vi "WebView2 Viewer.vi"(2 "ProjectRef":refnum<vi>, 4 "Extra Scripts":string, 5 "FileDependency In":map{path, T1}(c390), 6 "Options":string, 7 "OpenWebBrowser(False)":bool, 8 "error in":errorcluster, 9 "Embedd VISJS Librarya in HTMl File(False)":bool, 10 "HTMLFilePath":path, 11 "LibraryDependency":map{path, T3}(c390)) -> (0 "error out":errorcluster, 3 "HTMLFileContent":string)   [LabVIEW 2020, in "WebView2-Viewer.lvlib"] (continued)
break}for(C||(C={id:t.id},g.node&&(C.attr=Yv(C.attr,g.node))),A=I.length-1;A>=0;A--){var o,n=I[A];n.nodes||(n.nodes=[]),-1===Xc(o=n.nodes).call(o,C)&&n.nodes.push(C)}t.attr&&(C.attr=Yv(C.attr,t.attr))}function Uv(g,t){if(g.edges||(g.edges=[]),g.edges.push(t),g.edge){var A=Yv({},g.edge);t.attr=Yv(A,t.attr)}}function _v(g,t,A,e,C){var I={from:t,to:A,type:e};return g.edge&&(I.attr=Yv({},g.edge)),I.attr=Yv(I.attr||{},C),null!=C&&C.hasOwnProperty(\"arrows\")&&null!=C.arrows&&(I.arrows={to:{enabled:!0,type:C.arrows.type}},C.arrows=null),I}function Kv(){for(Gv=Mv.NULL,Fv=\"\";\" \"===Zv||\"\\t\"===Zv||\"\\n\"===Zv||\"\\r\"===Zv;)jv();do{var g=!1;if(\"#\"===Zv){for(var t=Sv-1;\" \"===zv.charAt(t)||\"\\t\"===zv.charAt(t);)t--;if(\"\\n\"===zv.charAt(t)||\"\"===zv.charAt(t)){for(;\"\"!=Zv&&\"\\n\"!=Zv;)jv();g=!0}}if(\"/\"===Zv&&\"/\"===Lv()){for(;\"\"!=Zv&&\"\\n\"!=Zv;)jv();g=!0}if(\"/\"===Zv&&\"*\"===Lv()){for(;\"\"!=Zv;){if(\"*\"===Zv&&\"/\"===Lv()){jv(),jv();break}jv()}g=!0}for(;\" \"===Zv||\"\\t\"===Zv||\"\\n\"===Zv||\"\\r\"===Zv;)jv()}while(g);if(\"\"!==Zv){var A=Zv+Lv();if(Bv[A])return Gv=Mv.DELIMITER,Fv=A,jv(),void jv();if(Bv[Zv])return Gv=Mv.DELIMITER,Fv=Zv,void jv();if(Vv(Zv)||\"-\"===Zv){for(Fv+=Zv,jv();Vv(Zv);)Fv+=Zv,jv();return\"false\"===Fv?Fv=!1:\"true\"===Fv?Fv=!0:isNaN(Number(Fv))||(Fv=Number(Fv)),void(Gv=Mv.IDENTIFIER)}if('\"'===Zv){for(jv();\"\"!=Zv&&('\"'!=Zv||'\"'===Zv&&'\"'===Lv());)'\"'===Zv?(Fv+=Zv,jv()):\"\\\\\"===Zv&&\"n\"===Lv()?(Fv+=\"\\n\",jv()):Fv+=Zv,jv();if('\"'!=Zv)throw gy('End of string \" expected');return jv(),void(Gv=Mv.IDENTIFIER)}for(Gv=Mv.UNKNOWN;\"\"!=Zv;)Fv+=Zv,jv();throw new SyntaxError('Syntax error in part \"'+ty(Fv,30)+'\"')}Gv=Mv.DELIMITER}function Hv(g){for(;\"\"!==Fv&&\"}\"!=Fv;)Xv(g),\";\"===Fv&&Kv()}function Xv(g){var t=Jv(g);if(t)qv(g,t);else{var A=function(g){if(\"node\"===Fv)return Kv(),g.node=$v(),\"node\";if(\"edge\"===Fv)return Kv(),g.edge=$v(),\"edge\";if(\"graph\"===Fv)return Kv(),g.graph=$v(),\"graph\";return null}(g);if(!A){if(Gv!=Mv.IDENTIFIER)throw gy(\"Identifier expected\");var e=Fv;if(Kv(),\"=\"===Fv){if(Kv(),Gv!=Mv.IDENTIFIER)throw gy(\"Identifier expected\");g[e]=Fv,Kv()}else!function(g,t){var A={id:t},e=$v();e&&(A.attr=e);Qv(g,A),qv(g,t)}(g,e)}}}function Jv(g){var t=null;if(\"subgraph\"===Fv&&((t={}).type=\"subgraph\",Kv(),Gv===Mv.IDENTIFIER&&(t.id=Fv,Kv())),\"{\"===Fv){if(Kv(),t||(t={}),t.parent=g,t.node=g.node,t.edge=g.edge,t.graph=g.graph,Hv(t),\"}\"!=Fv)throw gy(\"Angle bracket } expected\");Kv(),delete t.node,delete t.edge,delete t.graph,delete t.parent,g.subgraphs||(g.subgraphs=[]),g.subgraphs.push(t)}return t}function qv(g,t){for(;\"->\"===Fv||\"--\"===Fv;){var A,e=Fv;Kv();var C=Jv(g);if(C)A=C;else{if(Gv!=Mv.IDENTIFIER)throw gy(\"Identifier or subgraph expected\");Qv(g,{id:A=Fv}),Kv()}Uv(g,_v(g,t,A,e,$v())),t=A}}function $v(){for(var g,t,A=null,e={dashed:!0,solid:!1,dotted:[1,5]},C={dot:\"circle\",box:\"box\",crow:\"crow\",curve:\"curve\",icurve:\"inv_curve\",normal:\"triangle\",inv:\"inv_triangle\",diamond:\"diamond\",tee:\"bar\",vee:\"vee\"},I=new Array,i=new Array;\"[\"===Fv;){for(Kv(),A={};\"\"!==Fv&&\"]\"!=Fv;){if(Gv!=Mv.IDENTIFIER)throw gy(\"Attribute name expected\");var o=Fv;if(Kv(),\"=\"!=Fv)throw gy(\"Equal sign = expected\");if(Kv(),Gv!=Mv.IDENTIFIER)throw gy(\"Attribute value expected\");var n=Fv;\"style\"===o&&(n=e[n]),\"arrowhead\"===o&&(o=\"arrows\",n={to:{enabled:!0,type:C[n]}}),\"arrowtail\"===o&&(o=\"arrows\",n={from:{enabled:!0,type:C[n]}}),I.push({attr:A,name:o,value:n}),i.push(o),Kv(),\",\"==Fv&&Kv()}if(\"]\"!=Fv)throw gy(\"Bracket ] expected\");Kv()}if(Ic(i).call(i,\"dir\")){var r={arrows:{}};for(g=0;g<I.length;g++)if(\"arrows\"===I[g].name)if(null!=I[g].value.to)r.arrows.to=g;else{if(null==I[g].value.from)throw gy(\"Invalid value of arrows\");r.arrows.from=g}else\"dir\"===I[g].name&&(r.dir=g);var s,a,d=I[r.dir].value;if(!Ic(i).call(i,\"arrows\"))if(\"both\"===d)I.push({attr:I[r.dir].attr,name:\"arrows\",value:{to:{enabled:!0}}}),r.arrows.to=I.length-1,I.push({attr:I[r.dir].attr,name:\"arrows\",value:{from:{enabled:!0}}}),r.arrows.from=I.length-1;else if(\"forward\"===d)I.push({attr:I[r.dir].attr,name:\"arrows\",value:{to:{enabled:!0}}}),r.arrows.to=I.length-1;else if(\"back\"===d)I.push({attr:I[r.dir].attr,name:\"arrows\",value:{from:{enabled:!0}}}),r.arrows.from=I.length-1;else{if(\"none\"!==d)throw gy('Invalid dir type \"'+d+'\"');I.push({attr:I[r.dir].attr,name:\"arrows\",value:\"\"}),r.arrows.to=I.length-1}if(\"both\"===d)r.arrows.to&&r.arrows.from?(a=I[r.arrows.to].value.to.type,s=I[r.arrows.from].value.from.type,I[r.arrows.to]={attr:I[r.arrows.to].attr,name:I[r.arrows.to].name,value:{to:{enabled:!0,type:a},from:{enabled:!0,type:s}}},Zl(I).call(I,r.arrows.from,1)):r.arrows.to?(a=I[r.arrows.to].value.to.type,s=\"arrow\",I[r.arrows.to]={attr:I[r.arrows.to].attr,name:I[r.arrows.to].name,value:{to:{enabled:!0,type:a},from:{enabled:!0,type:s}}}):r.arrows.from&&(a=\"arrow\",s=I[r.arrows.from].value.from.type,I[r.arrows.from]={attr:I[r.arrows.from].attr,name:I[r.arrows.from].name,value:{to:{enabled:!0,type:a},from:{enabled:!0,type:s}}});else if(\"back\"===d)r.arrows.to&&r.arrows.from?(a=\"\",s=I[r.arrows.from].value.from.type,I[r.arrows.from]={attr:I[r.arrows.from].attr,name:I[r.arrows.from].name,value:{to:{enabled:!0,type:a},from:{enabled:!0,type:s}}}):r.arrows.to?(a=\"\",s=\"arrow\",r.arrows.from=r.arrows.to,I[r.arrows.from]={attr:I[r.arrows.from].attr,name:I[r.arrows.from].name,value:{to:{enabled:!0,type:a},from:{enabled:!0,type:s}}}):r.arrows.from&&(a=\"\",s=I[r.arrows.from].value.from.type,I[r.arrows.to]={attr:I[r.arrows.from].attr,name:I[r.arrows.from].name,value:{to:{enabled:!0,type:a},from:{enabled:!0,type:s}}}),I[r.arrows.from]={attr:I[r.arrows.from].attr,name:I[r.arrows.from].name,value:{from:{enabled:!0,type:I[r.arrows.from].value.from.type}}};else if(\"none\"===d){var h;I[h=r.arrows.to?r.arrows.to:r.arrows.from]={attr:I[h].attr,name:I[h].name,value:\"\"}}else{if(\"forward\"!==d)throw gy('Invalid dir type \"'+d+'\"');r.arrows.to&&r.arrows.from||r.arrows.to?(a=I[r.arrows.to].value.to.type,s=\"\",I[r.arrows.to]={attr:I[r.arrows.to].attr,name:I[r.arrows.to].name,value:{to:{enabled:!0,type:a},from:{enabled:!0,type:s}}}):r.arrows.from&&(a=\"arrow\",s=\"\",r.arrows.to=r.arrows.from,I[r.arrows.to]={attr:I[r.arrows.to].attr,name:I[r.arrows.to].name,value:{to:{enabled:!0,type:a},from:{enabled:!0,type:s}}}),I[r.arrows.to]={attr:I[r.arrows.to].attr,name:I[r.arrows.to].name,value:{to:{enabled:!0,type:I[r.arrows.to].value.to.type}}}}Zl(I).call(I,r.dir,1)}if(Ic(i).call(i,\"penwidth\")){var l=[];for(t=I.length,g=0;g<t;g++)\"width\"!==I[g].name&&(\"penwidth\"===I[g].name&&(I[g].name=\"width\"),l.push(I[g]));I=l}for(t=I.length,g=0;g<t;g++)Wv(I[g].attr,I[g].name,I[g].value);return A}function gy(g){return new SyntaxError(g+', got \"'+ty(Fv,30)+'\" (char '+Sv+\")\")}function ty(g,t){return g.length<=t?g:g.substr(0,27)+\"...\"}function Ay(g,t,A){for(var e=t.split(\".\"),C=e.pop(),I=g,i=0;i<e.length;i++){var o=e[i];o in I||(I[o]={}),I=I[o]}return I[C]=A,g}function ey(g,t){var A={};for(var e in g)if(g.hasOwnProperty(e)){var C=t[e];Rh(C)?Cl(C).call(C,(function(t){Ay(A,t,g[e])})):Ay(A,\"string\"==typeof C?C:e,g[e])}return A}function Cy(g){var t,A=Nv(g),e={nodes:[],edges:[],options:{}};A.nodes&&Cl(t=A.nodes).call(t,(function(g){var t={id:g.id,label:String(g.label||g.id)};Yv(t,ey(g.attr,Rv)),t.image&&(t.shape=\"image\"),e.nodes.push(t)}));if(A.edges){var C,I=function(g){var t={from:g.from,to:g.to};return Yv(t,ey(g.attr,Pv)),null==t.arrows&&\"->\"===g.type&&(t.arrows=\"to\"),t};Cl(C=A.edges).call(C,(function(g){var t,A,C,i,o,n,r;(t=g.from instanceof Object?g.from.nodes:{id:g.from},A=g.to instanceof Object?g.to.nodes:{id:g.to},g.from instanceof Object&&g.from.edges)&&Cl(C=g.from.edges).call(C,(function(g){var t=I(g);e.edges.push(t)}));(o=A,n=function(t,A){var C=_v(e,t.id,A.id,g.type,g.attr),i=I(C);e.edges.push(i)},Rh(i=t)?Cl(i).call(i,(function(g){Rh(o)?Cl(o).call(o,(function(t){n(g,t)})):n(g,o)})):Rh(o)?Cl(o).call(o,(function(g){n(i,g)})):n(i,o),g.to instanceof Object&&g.to.edges)&&Cl(r=g.to.edges).call(r,(function(g){var t=I(g);e.edges.push(t)}))}))}return A.attr&&(e.options=A.attr),e}var Iy=Object.freeze({__proto__:null,DOTToGraph:Cy,parseDOT:Nv});function iy(g,t){var A,e={edges:{inheritColor:!1},nodes:{fixed:!1,parseColor:!1}};null!=t&&(null!=t.fixed&&(e.nodes.fixed=t.fixed),null!=t.parseColor&&(e.nodes.parseColor=t.parseColor),null!=t.inheritColor&&(e.edges.inheritColor=t.inheritColor));var C=g.edges,I=Fh(C).call(C,(function(g){var t={from:g.source,id:g.id,to:g.target};return null!=g.attributes&&(t.attributes=g.attributes),null!=g.label&&(t.label=g.label),null!=g.attributes&&null!=g.attributes.title&&(t.title=g.attributes.title),\"Directed\"===g.type&&(t.arrows=\"to\"),g.color&&!1===e.edges.inheritColor&&(t.color=g.color),t}));return{nodes:Fh(A=g.nodes).call(A,(function(g){var t={id:g.id,fixed:e.nodes.fixed&&null!=g.x&&null!=g.y};return null!=g.attributes&&(t.attributes=g.attributes),null!=g.label&&(t.label=g.label),null!=g.size&&(t.size=g.size),null!=g.attributes&&null!=g.attributes.title&&(t.title=g.attributes.title),null!=g.title&&(t.title=g.title),null!=g.x&&(t.x=g.x),null!=g.y&&(t.y=g.y),null!=g.color&&(!0===e.nodes.parseColor?t.color=g.color:t.color={background:g.color,border:g.color,highlight:{background:g.color,border:g.color},hover:{background:g.color,border:g.color}}),t})),edges:I}}var oy=Object.freeze({__proto__:null,parseGephi:iy}),ny=Object.freeze({__proto__:null,cn:{addDescription:\"???????????\",addEdge:\"?????\",addNode:\"????\",back:\"??\",close:\"??\",createEdgeError:\"????????????\",del:\"????\",deleteClusterError:\"???????\",edgeDescription:\"??????????????????????????\",edit:\"??\",editClusterError:\"???????\",editEdge:\"?????\",editEdgeDescription:\"??????????????????\",editNode:\"????\"},cs:{addDescription:\"Kluknutím do prázdného prostoru mužete pridat nový vrchol.\",addEdge:\"Pridat hranu\",addNode:\"Pridat vrchol\",back:\"Zpet\",close:\"Zavrít\",createEdgeError:\"Nelze pripojit hranu ke shluku.\",del:\"Smazat výber\",deleteClusterError:\"Nelze mazat shluky.\",edgeDescription:\"Pretažením z jednoho vrcholu do druhého mužete spojit tyto vrcholy novou hranou.\",edit:\"Upravit\",editClusterError:\"Nelze upravovat shluky.\",editEdge:\"Upravit hranu\",editEdgeDescription:\"Pretažením kontrolního vrcholu hrany ji mužete pripojit k jinému vrcholu.\",editNode:\"Upravit vrchol\"},de:{addDescription:\"Klicke auf eine freie Stelle, um einen neuen Knoten zu plazieren.\",addEdge:\"Kante hinzufügen\",addNode:\"Knoten hinzufügen\",back:\"Zurück\",close:\"Schließen\",createEdgeError:\"Es ist nicht möglich, Kanten mit Clustern zu verbinden.\",del:\"Lösche Auswahl\",deleteClusterError:\"Cluster können nicht gelöscht werden.\",edgeDescription:\"Klicke auf einen Knoten und ziehe die Kante zu einem anderen Knoten, um diese zu verbinden.\",edit:\"Editieren\",editClusterError:\"Cluster können nicht editiert werden.\",editEdge:\"Kante editieren\",editEdgeDescription:\"Klicke auf die Verbindungspunkte und ziehe diese auf einen Knoten, um sie zu verbinden.\",editNode:\"Knoten editieren\"},en:{addDescription:\"Click in an empty space to place a new node.\",addEdge:\"Add Edge\",addNode:\"Add Node\",back:\"Back\",close:\"Close\",createEdgeError:\"Cannot link edges to a cluster.\",del:\"Delete selected\",deleteClusterError:\"Clusters cannot be deleted.\",edgeDescription:\"Click on a node and drag the edge to another node to connect them.\",edit:\"Edit\",editClusterError:\"Clusters cannot be edited.\",editEdge:\"Edit Edge\",editEdgeDescription:\"Click on the control points and drag them to a node to connect to it.\",editNode:\"Edit Node\"},es:{addDescription:\"Haga clic en un lugar vacío para colocar un nuevo nodo.\",addEdge:\"Añadir arista\",addNode:\"Añadir nodo\",back:\"Atrás\",close:\"Cerrar\",createEdgeError:\"No se puede conectar una arista a un grupo.\",del:\"Eliminar selección\",deleteClusterError:\"No es posible eliminar grupos.\",edgeDescription:\"Haga clic en un nodo y arrastre la arista hacia otro nodo para conectarlos.\",edit:\"Editar\",editClusterError:\"No es posible editar grupos.\",editEdge:\"Editar arista\",editEdgeDescription:\"Haga clic en un punto de control y arrastrelo a un nodo para conectarlo.\",editNode:\"Editar nodo\"},fr:{addDescription:\"Cliquez dans un endroit vide pour placer un nœud.\",addEdge:\"Ajouter un lien\",addNode:\"Ajouter un nœud\",back:\"Retour\",close:\"Fermer\",createEdgeError:\"Impossible de créer un lien vers un cluster.\",del:\"Effacer la sélection\",deleteClusterError:\"Les clusters ne peuvent pas être effacés.\",edgeDescription:\"Cliquez sur un nœud et glissez le lien vers un autre nœud pour les connecter.\",edit:\"Éditer\",editClusterError:\"Les clusters ne peuvent pas être édités.\",editEdge:\"Éditer le lien\",editEdgeDescription:\"Cliquez sur les points de contrôle et glissez-les pour connecter un nœud.\",editNode:\"Éditer le nœud\"},it:{addDescription:\"Clicca per aggiungere un nuovo nodo\",addEdge:\"Aggiungi un vertice\",addNode:\"Aggiungi un nodo\",back:\"Indietro\",close:\"Chiudere\",createEdgeError:\"Non si possono collegare vertici ad un cluster\",del:\"Cancella la selezione\",deleteClusterError:\"I cluster non possono essere cancellati\",edgeDescription:\"Clicca su un nodo e trascinalo ad un altro nodo per connetterli.\",edit:\"Modifica\",editClusterError:\"I clusters non possono essere modificati.\",editEdge:\"Modifica il vertice\",editEdgeDescription:\"Clicca sui Punti di controllo e trascinali ad un nodo per connetterli.\",editNode:\"Modifica il nodo\"},nl:{addDescription:\"Klik op een leeg gebied om een nieuwe node te maken.\",addEdge:\"Link toevoegen\",addNode:\"Node toevoegen\",back:\"Terug\",close:\"Sluiten\",createEdgeError:\"Kan geen link maken naar een cluster.\",del:\"Selectie verwijderen\",deleteClusterError:\"Clusters kunnen niet worden verwijderd.\",edgeDescription:\"Klik op een node en sleep de link naar een andere node om ze te verbinden.\",edit:\"Wijzigen\",editClusterError:\"Clusters kunnen niet worden aangepast.\",editEdge:\"Link wijzigen\",editEdgeDescription:\"Klik op de verbindingspunten en sleep ze naar een node om daarmee te verbinden.\",editNode:\"Node wijzigen\"},pt:{addDescription:\"Clique em um espaço em branco para adicionar um novo nó\",addEdge:\"Adicionar aresta\",addNode:\"Adicionar nó\",back:\"Voltar\",close:\"Fechar\",createEdgeError:\"Não foi possível linkar arestas a um cluster.\",del:\"Remover selecionado\",deleteClusterError:\"Clusters não puderam ser removidos.\",edgeDescription:\"Clique em um nó e arraste a aresta até outro nó para conectá-los\",edit:\"Editar\",editClusterError:\"Clusters não puderam ser editados.\",editEdge:\"Editar aresta\",editEdgeDescription:\"Clique nos pontos de controle e os arraste para um nó para conectá-los\",editNode:\"Editar nó\"},ru:{addDescription:\"???????? ? ????????? ?????, ????? ???????? ????? ????.\",addEdge:\"???????? ?????\",addNode:\"???????? ????\",back:\"?????\",close:\"?????????\",createEdgeError:\"?????????? ????????? ????? ? ???????.\",del:\"??????? ?????????\",deleteClusterError:\"???????? ?? ????? ???? ???????\",edgeDescription:\"???????? ?? ???? ? ????????? ????? ? ??????? ????, ????? ????????? ??.\",edit:\"?????????????\",editClusterError:\"???????? ?????????? ??? ??????????????.\",editEdge:\"????????????? ?????\",editEdgeDescription:\"???????? ?? ??????????? ????? ? ?????????? ?? ? ????, ????? ???????????? ? ????.\",editNode:\"????????????? ????\"},uk:{addDescription:\"K??????? ?? ?????? ?????, ??? ?????? ????? ?????.\",addEdge:\"?????? ????\",addNode:\"?????? ?????\",back:\"?????\",close:\"???????\",createEdgeError:\"?? ??????? ??'?????? ???? ? ?????.\",del:\"???????? ??????\",deleteClusterError:\"????? ?? ?????? ???? ????????.\",edgeDescription:\"???????? ?? ????? ? ??????????? ???? ?? ?????? ?????, ??? ?? ?'??????.\",edit:\"??????????\",editClusterError:\"????? ?????????? ??? ???????????.\",editEdge:\"?????????? ????\",editEdgeDescription:\"???????? ?? ?????????? ????? ? ??????????? ?? ? ?????, ??? ???????????? ?? ?????.\",editNode:\"?????????? ?????\"}});var ry=function(){function g(){cn(this,g),this.NUM_ITERATIONS=4,this.image=new Image,this.canvas=document.createElement(\"canvas\")}return kd(g,[{key:\"init\",value:function(){if(!this.initialized()){this.src=this.image.src;var g=this.image.width,t=this.image.height;this.width=g,this.height=t;var A=Math.floor(t/2),e=Math.floor(t/4),C=Math.floor(t/8),I=Math.floor(t/16),i=Math.floor(g/2),o=Math.floor(g/4),n=Math.floor(g/8),r=Math.floor(g/16);this.canvas.width=3*o,this.canvas.height=A,this.coordinates=[[0,0,i,A],[i,0,o,e],[i,e,n,C],[5*n,e,r,I]],this._fillMipMap()}}},{key:\"initialized\",value:function(){return void 0!==this.coordinates}},{key:\"_fillMipMap\",value:function(){var g=this.canvas.getContext(\"2d\"),t=this.coordinates[0];g.drawImage(this.image,t[0],t[1],t[2],t[3]);for(var A=1;A<this.NUM_ITERATIONS;A++){var e=this.coordinates[A-1],C=this.coordinates[A];g.drawImage(this.canvas,e[0],e[1],e[2],e[3],C[0],C[1],C[2],C[3])}}},{key:\"drawImageAtPosition\",value:function(g,t,A,e,C,I){if(this.initialized())if(t>2){t*=.5;for(var i=0;t>2&&i<this.NUM_ITERATIONS;)t*=.5,i+=1;i>=this.NUM_ITERATIONS&&(i=this.NUM_ITERATIONS-1);var o=this.coordinates[i];g.drawImage(this.canvas,o[0],o[1],o[2],o[3],A,e,C,I)}else g.drawImage(this.image,A,e,C,I)}}]),g}(),sy=function(){function g(t){cn(this,g),this.images={},this.imageBroken={},this.callback=t}return kd(g,[{key:\"_tryloadBrokenUrl\",value:function(g,t,A){void 0!==g&&void 0!==A&&(void 0!==t?(A.image.onerror=function(){console.error(\"Could not load brokenImage:\",t)},A.image.src=t):console.warn(\"No broken url image defined\"))}},{key:\"_redrawWithImage\",value:function(g){this.callback&&this.callback(g)}},{key:\"load\",value:function(g,t){var A=this,e=this.images[g];if(e)return e;var C=new ry;return this.images[g]=C,C.image.onload=function(){A._fixImageCoordinates(C.image),C.init(),A._redrawWithImage(C)},C.image.onerror=function(){console.error(\"Could not load image:\",g),A._tryloadBrokenUrl(g,t,C)},C.image.src=g,C}},{key:\"_fixImageCoordinates\",value:function(g){0===g.width&&(document.body.appendChild(g),g.width=g.offsetWidth,g.height=g.offsetHeight,document.body.removeChild(g))}}]),g}(),ay={exports:{}},dy=I((function(){if(\"function\"==typeof ArrayBuffer){var g=new ArrayBuffer(8);Object.isExtensible(g)&&Object.defineProperty(g,\"a\",{value:8})}})),hy=I,ly=gg,cy=y,uy=dy,py=Object.isExtensible,fy=hy((function(){py(1)}))||uy?function(g){return!!ly(g)&&((!uy||\"ArrayBuffer\"!==cy(g))&&(!py||py(g)))}:py,vy=!I((function(){return Object.isExtensible(Object.preventExtensions({}))})),yy=TA,my=u,by=UA,wy=gg,ky=qg,xy=Jt.f,Ey=gr,Oy=er,Ty=fy,Dy=vy,Ny=!1,Ry=et(\"meta\"),Py=0,My=function(g){xy(g,Ry,{value:{objectID:\"O\"+Py++,weakData:{}}})},By=ay.exports={enable:function(){By.enable=function(){},Ny=!0;var g=Ey.f,t=my([].splice),A={};A[Ry]=1,g(A).length&&(Ey.f=function(A){for(var e=g(A),C=0,I=e.length;C<I;C++)if(e[C]===Ry){t(e,C,1);break}return e},yy({target:\"Object\",stat:!0,forced:!0},{getOwnPropertyNames:Oy.f}))},fastKey:function(g,t){if(!wy(g))return\"symbol\"==typeof g?g:(\"string\"==typeof g?\"S\":\"P\")+g;if(!ky(g,Ry)){if(!Ty(g))return\"F\";if(!t)return\"E\";My(g)}return g[Ry].objectID},getWeakData:function(g,t){if(!ky(g,Ry)){if(!Ty(g))return!0;if(!t)return!1;My(g)}return g[Ry].weakData},onFreeze:function(g){return Dy&&Ny&&Ty(g)&&!ky(g,Ry)&&My(g),g}};by[Ry]=!0;var zy=ay.exports,Sy=Xt,Zy=P,Fy=AA,Gy=Og,jy=Qi,Ly=jA,Vy=og,Yy=Oo,Wy=yo,Qy=Gi,Uy=TypeError,_y=function(g,t){this.stopped=g,this.result=t},Ky=_y.prototype,Hy=function(g,t,A){var e,C,I,i,o,n,r,s=A&&A.that,a=!(!A||!A.AS_ENTRIES),d=!(!A||!A.IS_RECORD),h=!(!A||!A.IS_ITERATOR),l=!(!A||!A.INTERRUPTED),c=Sy(t,s),u=function(g){return e&&Qy(e,\"normal\",g),new _y(!0,g)},p=function(g){return a?(Fy(g),l?c(g[0],g[1],u):c(g[0],g[1])):l?c(g,u):c(g)};
